vi "Grid.vi"() -> ()   [LabVIEW 2011]
panel:
  in  "End Example":bool
  in  "Grid (ON/OFF)":bool
  out "Waveform Chart":dbl(graph)=0.30467480593781415
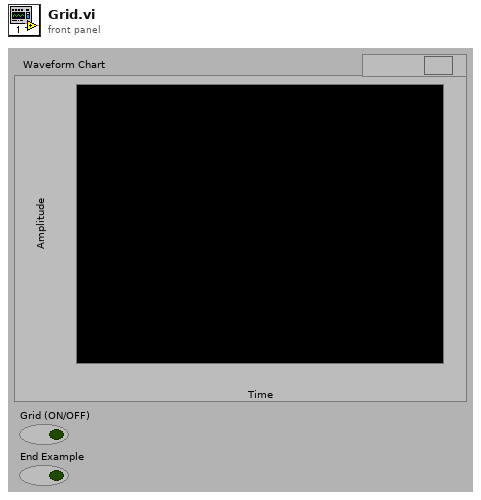
[diagram p1: front panel]
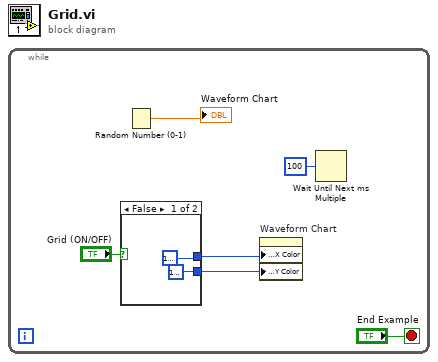
[diagram p0: block diagram]
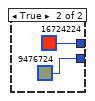
[diagram p2: hidden frame]
diagram:
  n1 = while {
    stop <- "End Example" stop-if-true
    n2 = case shown="False" "Grid (ON/OFF)" {
      tunnel: [u32 16777216 u32 16724224] -> w6
      tunnel: [u32 16777216 u32 9476724] -> w1
      frame False {
      }
      frame True {
      }
    }
    n3 = Random Number (0-1)() -> (number: 0 to 1=→"Waveform Chart":dbl)
    n4 = property on="Waveform Chart" class="WFChart (strict)"("Grid Colors:X Color"=w6, "Grid Colors:Y Color"=w1) -> ()  [unwired: 2 in, 2 out]
    n5 = Wait Until Next ms Multiple(millisecond multiple=u32 100) -> ()  [unwired: 1 out]
  }
